vi "HW_Calibration_fit.vi"(0 "coeff suffix":string, 5 "Fixed n (F)":bool, 6 "n input  (0.45)":dbl=0.45 format="%.4f", 7 "Point selector":cluster{"Y":dbl, "X":dbl, "switch":bool}[](array[cluster]) {"X" format="%.2f"; "Y" format="%.2f"}, 8 "Velocity":dbl[](array[numeric]) format="%.2f", 9 "HW voltage":dbl[](array[numeric]) format="%.2f") -> (1 "Calib const":string[][](array[string]), 2 "Calibration plot":cluster{cluster{dbl, "mse":dbl}[]}[](graph), 3 "Point selector":cluster{"Y":dbl, "X":dbl, "switch":bool}[](array[cluster]) {"X" format="%.2f"; "Y" format="%.2f"}, 4 "Coefficients":dbl[](array[numeric]) format="%.2f")   [LabVIEW 2010]
uses:
  Globals/Calib_global.vi
  <vilib>/Analysis/NI_AALPro.lvlib
  <vilib>/Analysis/NI_AALBase.lvlib
panel:
  in  "Type":cluster{"Y":dbl, "X":dbl, "switch":bool}={"Y"=10.144154930121, "X"=9.20412, "switch"=FALSE} {"X" format="%.2f"; "Y" format="%.2f"}
  # "This program fits a curve to a set of calibration  points as selected by the switches.   The program loops round to find the best value for n to give the minimum mean square error."
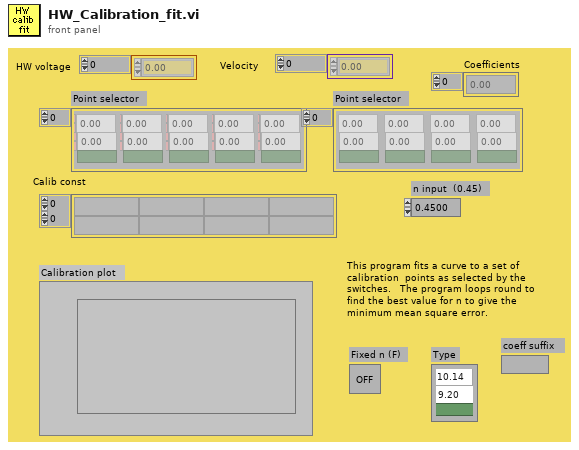
[diagram p1: front panel]
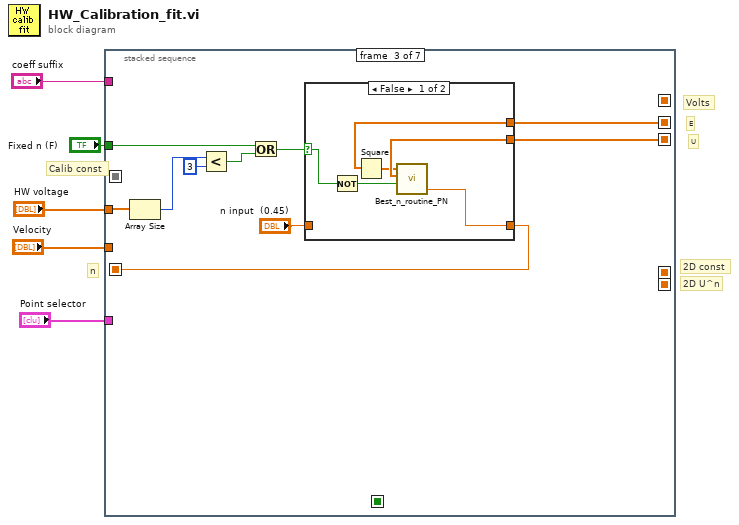
[diagram p0: block diagram]
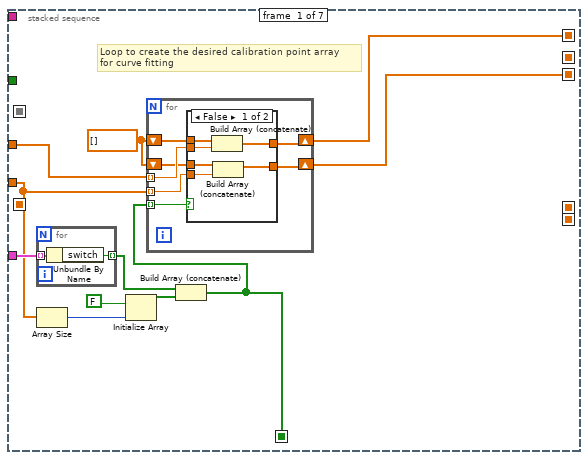
[diagram p2: hidden frame]
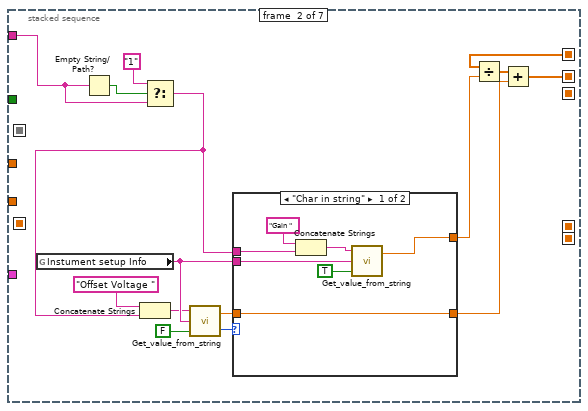
[diagram p4: hidden frame]
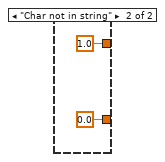
[diagram p5: hidden frame]
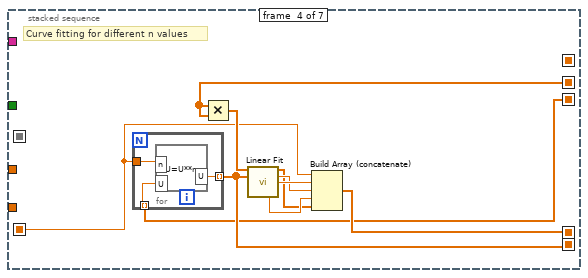
[diagram p7: hidden frame]
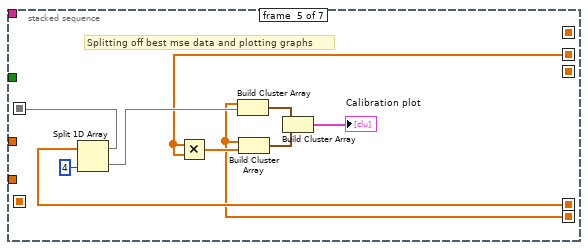
[diagram p8: hidden frame]
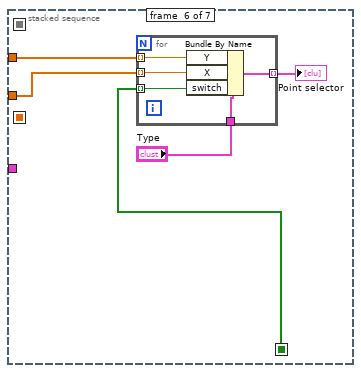
[diagram p9: hidden frame]
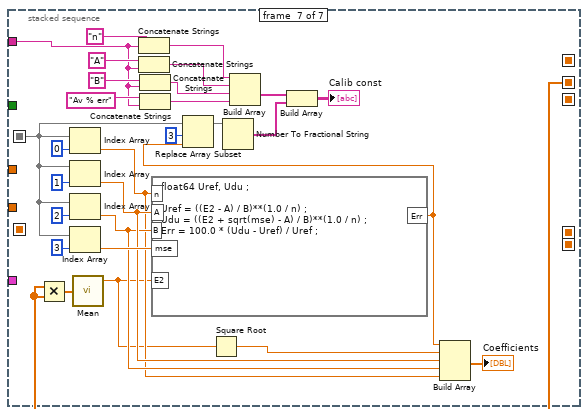
[diagram p10: hidden frame]
diagram:
  # "n"
  # "Volts"
  # "U"
  # "E"
  # "Calib const"
  # "2D U^n"
  # "2D const"
  n1 = stacked-sequence "E^2" {
    seq-local: [_ _ _ w82 _ _ _] -> [_ _ _ _ w88 _ _]
    seq-local: [_ _ _ w84 _ _ _] -> [_ _ _ _ w89 _ _]
    seq-local: [_ w40 _ _ _ _ _] -> [_ _ w67 w80 w91 _ w117]
    seq-local: [w7 _ _ _ _ _ _] -> [_ _ w66 w79 _ _ _]
    seq-local: [_ _ _ _ w93 _ _] -> [_ _ _ _ _ _ w131]
    seq-local: [w13 _ _ _ _ _ _] -> [_ _ _ _ _ w99 _]
    seq-local: [w6 _ _ _ _ _ _] -> [_ w43 _ _ _ _ _]
    seq-local: [_ _ w65 _ _ _ _] -> [_ _ _ w75 _ _ _]
    tunnel: "Velocity" -> [w10 _ _ _ _ w102 _]
    tunnel: "HW voltage" -> [w9 _ w63 _ _ w98 _]
    tunnel: "Point selector" -> [w16 _ _ _ _ _ _]
    tunnel: "coeff suffix" -> [_ w36 _ _ _ _ w108]
    tunnel: "Fixed n (F)" -> [_ _ w59 _ _ _ _]
    frame #0 {
      w8 = dbl[] []
      # "Loop to create the desired calibration point array\nfor curve fitting"
      n2 = for {
        tunnel: w16 -> [w18] mode=indexing
        tunnel: [w17] -> w15 mode=indexing
        n3 = Unbundle By Name(w18) -> ("switch"=w17:bool)
      }
      n4 = Array Size(array=w10) -> (size(s)=w11:i32)
      n5 = Initialize Array(FALSE, w11) -> (w14:bool[])
      n6 = Build Array (concatenate)(w15, w14) -> (w13:bool[])
      n7 = for {
        shift-right: [w19] -> w7
        shift-left: w8 -> [w21]
        shift-right: [w20] -> w6
        shift-left: w8 -> [w22]
        tunnel: w13 -> [w23] mode=indexing
        tunnel: w10 -> [w24] mode=indexing
        tunnel: w9 -> [w25] mode=indexing
        n8 = case shown="False" w23 {
          tunnel: [w26 w32] -> w19
          tunnel: [w27 w33] -> w20
          tunnel: w21 -> [w28 w32]
          tunnel: w22 -> [w29 w33]
          tunnel: w24 -> [w30 _]
          tunnel: w25 -> [w31 _]
          frame False {
            n9 = Build Array (concatenate)(w29, w31) -> (w27:dbl[])
            n10 = Build Array (concatenate)(w28, w30) -> (w26:dbl[])
          }
          frame True {
          }
        }
      }
    }
    frame #1 {
      n11 = global read "Calib_global.vi" "Instument setup Info"() -> (w45:string)
      n12 = Empty String/Path?(string/path=w36) -> (empty?=w37:bool)
      n13 = Select(t="1", s=w37, f=w36) -> (s? t:f=w34:string)
      n14 = Concatenate Strings("Offset Voltage ", w34) -> (w38:string)
      n15 = call "Get_value_from_string.vi"("Show Dialog?"=FALSE, "Input string"=w45, "Variable name"=w38) -> ("Status"=w47:enum16{"Char in string", "Char not in string"}, "Value"=w46:dbl)
      n16 = case shown="\"Char in string\"" w47 {
        tunnel: w45 -> [w55 _]
        tunnel: [w53 1.0 ("Value")] -> w44
        tunnel: w46 -> [w52 _]
        tunnel: [w52 0.0 ("Value")] -> w41
        tunnel: w34 -> [w49 _]
        frame "Char in string" {
          n17 = Concatenate Strings("Gain ", w49) -> (w51:string)
          n18 = call "Get_value_from_string.vi"("Show Dialog?"=TRUE, "Input string"=w55, "Variable name"=w51) -> ("Value"=w53:dbl)  [unwired: 1 out]
        }
        frame "Char not in string" {
        }
      }
      n19 = Divide(x=w43, y=w44) -> (x/y=w42:dbl[])
      n20 = Add(x=w42, y=w41) -> (x+y=w40:dbl[])
    }
    frame #2 {
      n21 = Array Size(array=w63) -> (size(s)=w62:i32)
      n22 = Less?(x=w62, y=3) -> (x < y?=w60:bool)
      n23 = Or(x=w59, y=w60) -> (x .or. y?=w58:bool)
      n24 = case shown="False" w58 {
        selector: w58 -> [w68 _]
        tunnel: w67 -> [w71 _]
        tunnel: w66 -> [w73 _]
        tunnel: [w72 w74] -> w65
        tunnel: "n input  (0.45)" -> [_ w74]
        frame False {
          n25 = Not(x=w68) -> (.not. x?=w69:bool)
          n26 = Square(x=w71) -> (x^2=w70:dbl[])
          n27 = call "Best_n_routine_PN.vi"("variable n?"=w69, "U"=w73, "E^2"=w70) -> ("n"=w72:dbl)  [unwired: 1 in, 2 out]
        }
        frame True {
        }
      }
    }
    frame #3 {
      # "Curve fitting for different n values"
      n28 = for {
        tunnel: [w86] -> w82 mode=indexing
        tunnel: w79 -> [w87] mode=indexing
        tunnel: w75 -> [w85]
        n29 = formula code="U=U**n;"("U"=w87, "n"=w85) -> ("U"=w86:dbl)
      }
      n30 = Multiply(x=w80, y=w80) -> (x*y=w81:dbl[])
      n31 = call <vilib>:"Linear Fit.vi"("Y"=w81, "X"=w82) -> ("Best Linear Fit"=w76:dbl[], "slope"=w77:dbl, "intercept"=w78:dbl, "residue"=w83:dbl)  [unwired: 4 in, 6 out]
      n32 = Build Array (concatenate)(w75, w78, w77, w83, w76) -> (w84:dbl[])
    }
    frame #4 {
      # "Splitting off best mse data and plotting graphs"
      n33 = Split 1D Array(array=w89, index=4) -> (first subarray=w93:dbl[], second subarray=w94:dbl[])
      n34 = Multiply(x=w91, y=w91) -> (x*y=w90:dbl[])
      n35 = Build Cluster Array(w88, w94) -> (w92:cluster{"U":dbl, "Numeric":dbl}[])
      n36 = Build Cluster Array(w88, w90) -> (w97:cluster{"U":dbl, dbl}[])
      n37 = Build Cluster Array(w92, w97) -> (→"Calibration plot":cluster{cluster{"U":dbl, "Numeric":dbl}[]}[])
    }
    frame #5 {
      n38 = for {
        tunnel: w98 -> [w107] mode=indexing
        tunnel: w102 -> [w106] mode=indexing
        tunnel: [w105] -> w101 mode=indexing
        tunnel: "Type" -> [w104]
        tunnel: w99 -> [w103] mode=indexing
        n39 = Bundle By Name(cluster=w104, "Y"=w107, "X"=w106, "switch"=w103) -> (w105:cluster{"Y":dbl, "X":dbl, "switch":bool})
      }
      "Point selector" <- w101
    }
    frame #6 {
      n40 = Multiply(x=w117, y=w117) -> (x*y=w116:dbl[])
      n41 = Index Array(array=w131, index=0) -> (element=w113:dbl)
      n42 = Index Array(array=w131, index=1) -> (element=w115:dbl)
      n43 = Index Array(array=w131, index=2) -> (element=w114:dbl)
      n44 = Index Array(array=w131, index=3) -> (element=w132:dbl)
      n45 = call <vilib>:"Mean.vi"("X"=w116) -> ("mean"=w110:dbl)  [unwired: 1 out]
      n46 = Concatenate Strings("n", w108) -> (w121:string)
      n47 = Concatenate Strings("A", w108) -> (w120:string)
      n48 = Concatenate Strings("B", w108) -> (w119:string)
      n49 = Concatenate Strings("Av % err", w108) -> (w118:string)
      n50 = formula code="float64 Uref, Udu ;\n\nUref = ((E2 - A) / B)**(1.0 / n) ;\nUdu = ((E2 + sqrt(mse) - A) / B)**(1.0 / n) ;\nErr = 100.0 * (Udu - Uref) / Uref ;"("n"=w113, "A"=w115, "B"=w114, "mse"=w132, "E2"=w110) -> ("Err"=w111:dbl)
      n51 = Replace Array Subset(array=w131, new element=w111, index=3) -> (w129:dbl[])
      n52 = Square Root(x=w110) -> (sqrt(x)=w109:dbl)
      n53 = Number To Fractional String(number=w129) -> (F-format string=w128:string[])  [unwired: 3 out]
      n54 = Build Array(w121, w120, w119, w118) -> (w127:string[])
      n55 = Build Array(w127, w128) -> (→"Calib const":string[][])
      n56 = Build Array(w111, w109, w115, w114, w113) -> (→"Coefficients":dbl[])
    }
  }
